vi "GA_Global.vi"() -> ()   [LabVIEW 2018]
uses:
  Control/GA_parameter.ctl
panel:
  out "pop(500*20)":i32[][](array[numeric])
  out "city_position(20*2)":dbl[][](array[numeric])
  in  "Parameter":T1
  # "20 city"
  # "500 ¤H"
  # "X"
  # "Y"
  # "City"
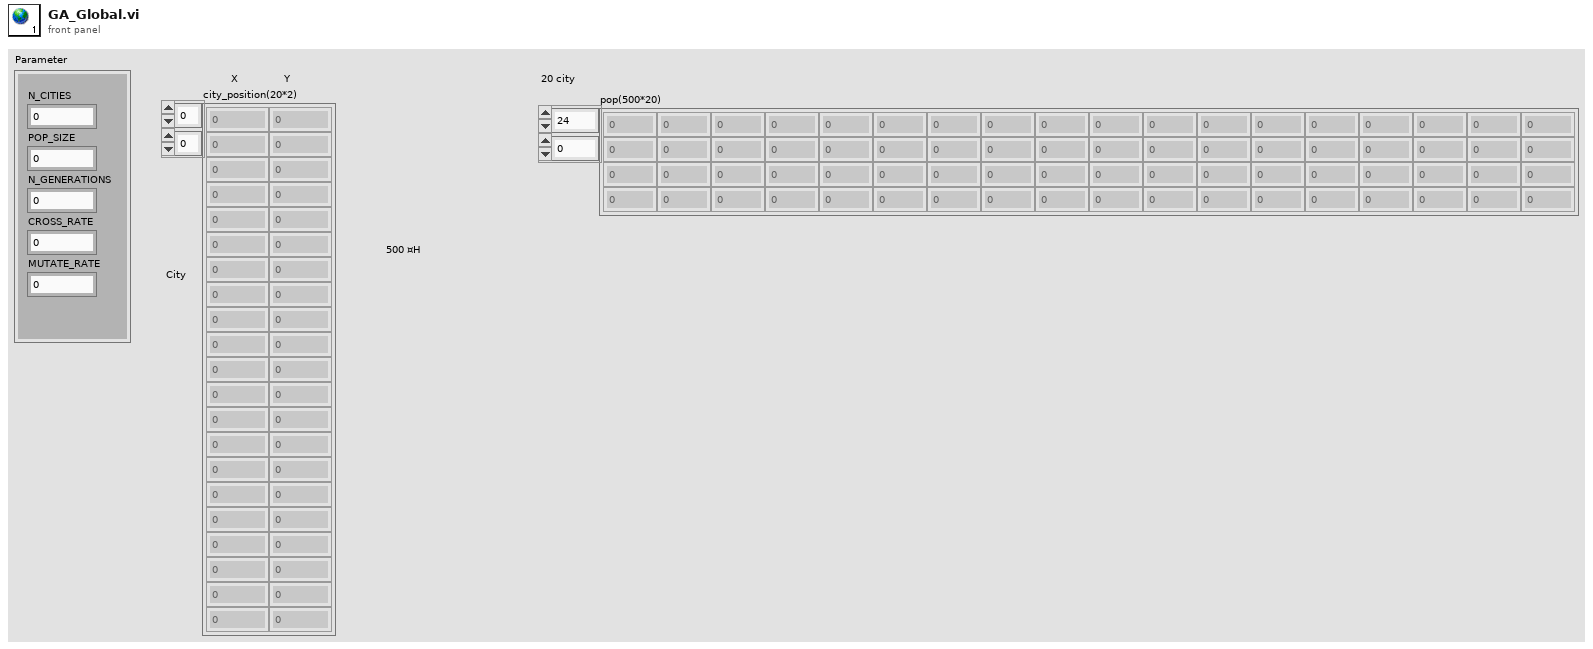
[diagram p1: front panel]
types:
  T1 = typedef "GA_parameter.ctl" = cluster{"N_CITIES":i32, "POP_SIZE":i32, "N_GENERATIONS":i32, "CROSS_RATE":dbl, "MUTATE_RATE":dbl}
diagram:
